vi "AngularDistance.vi"(1 "Goal Angle (deg) [0,360]":dbl format="%#_13g", 2 "Current Angle (deg) [-Inf,+Inf]":dbl format="%#_13g") -> (0 "Signed Angular Distance (deg)":dbl format="%_4g")   [LabVIEW 2019]
doc: "Calculates the signed angular distance from the Current Angle to the Goal Angle. The Goal Angle must be on [0,360] while the Current angle can be on [-Inf,+Inf]."
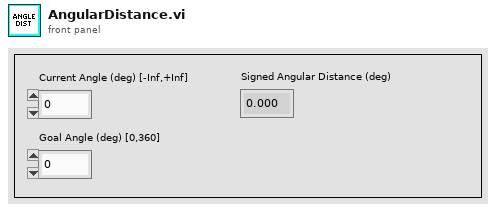
[diagram p1: front panel]
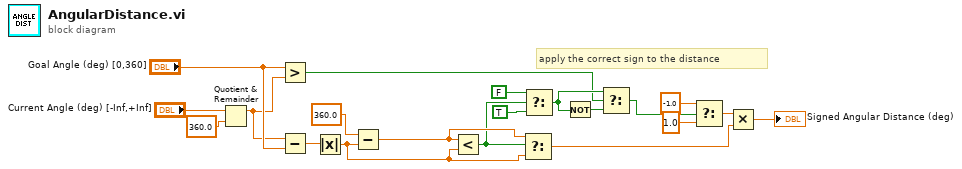
[diagram p0: block diagram]
diagram:
  # "apply the correct sign to the distance"
  n1 = Quotient & Remainder(x="Current Angle (deg) [-Inf,+Inf]", y=360.0) -> (x-y*floor(x/y)=w15:dbl)  [unwired: 1 out]
  n2 = Greater?(x="Goal Angle (deg) [0,360]", y=w15) -> (0:w8:bool)
  n3 = Subtract(x=w15, y="Goal Angle (deg) [0,360]") -> (x-y=w18:dbl)
  n4 = Absolute Value(x=w18) -> (abs(x)=w13:dbl)
  n5 = Subtract(x=360.0, y=w13) -> (x-y=w14:dbl)
  n6 = Less?(x=w14, y=w13) -> (x < y?=w12:bool)
  n7 = Select(t=w14, s=w12, f=w13) -> (s? t:f=w2:dbl)
  n8 = Select(t=FALSE, s=w12, f=TRUE) -> (s? t:f=w9:bool)
  n9 = Not(x=w9) -> (.not. x?=w7:bool)
  n10 = Select(t=w9, s=w8, f=w7) -> (s? t:f=w6:bool)
  n11 = Select(t=-1.0, s=w6, f=1.0) -> (s? t:f=w3:dbl)
  n12 = Multiply(x=w3, y=w2) -> (x*y=→"Signed Angular Distance (deg)":dbl)
